vi "updateNonRf.vi"(8 "error in (no error)":errorcluster, 11 "StaticOutputEditor in":refnum<class "StaticOutputEditor.lvclass">) -> (0 "error out":errorcluster, 3 "StaticOutputEditor out":refnum<class "StaticOutputEditor.lvclass">)   [LabVIEW 2011, in "Views.lvlib" / "ScriptEditor.lvlib" / "StaticOutputEditor.lvclass"]
uses:
  StaticOutputEditor.lvclass
  StaticOutputEditor.lvclass/StaticOutputEditor.ctl
  Hal/HWController/HWControllerEvents/HWControllerEvents.lvclass
  Tools/DatabaseHelpers/Database Objects/ChannelArray/ChannelArray.lvclass
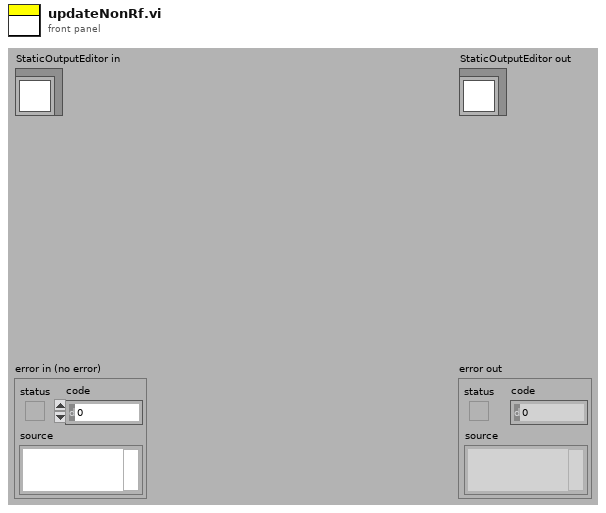
[diagram p1: front panel]
types:
  T1 = enum16{"start", "stop", "statusInquiry", "configure", "resetError", "resourcesInquiry", "reserveResources", "initialise", "resetAllChannels", "staticUpdate", "close", "HWStatus", "error", "resourcesAvailable", "resourcesReserved", "compilerError", "compiledScript", "compilingScript", "runScript", "configureCompiledScript"}
  T2 = cluster{"channelName":string, "value":string, "freq":string, "phase":string}[]
  T3 = cluster{"channelName":string, "value":string, "freq":string, "phase":string}
  T4 = cluster{"incomingEventTypes":cluster{"start":cluster{"Boolean":bool}, "stop":cluster{"Boolean":bool}, "statusInquiry":cluster{"Boolean":bool}, "configure":cluster{"DPScriptPath":path, "TimeStamp":string, "HWLoop?":bool}, "resetError":cluster{"Boolean":bool}, "resourcesInquiry":cluster{"Boolean":bool}, "reserveResources":cluster{"HWList":string[]}, "initialise":cluster{"HWList":string[]}, "close":cluster{"Boolean":bool}, "resetAllChannels":cluster{"Boolean":bool}, "staticChannelUpdate":cluster{"channel_address":string, "calibratedValue":dbl}, "runScript":cluster{"DPScriptPath":path, "TimeStamp":string, "HWLoop?":bool}, "compilingScript":cluster{"Path":path}, "compiledScript":cluster{"Path":path, "timeCompileAt":string}, "compilerError":cluster{"Path":path}, "configureCompiledScript":cluster{"DPScriptPath":path, "TimeStamp":string, "HWLoop?":bool, "CompiledScript":cluster{"ScriptListCompiler.lvclass":refnum<class "ScriptListCompiler.lvclass">, "aoChannels":refnum<class "AnalogOutput.lvclass">[], "doChannels":refnum<class "DigitalOutput.lvclass">[], "rfChannels":refnum<class "DDSOutput.lvclass">[]}}, "restartCompiler":cluster{"restart":bool}, "staticRfChannelUpdate":cluster{"channel_address":string, "Output":cluster{"Frequency(MHz)":dbl, "Amplitude":dbl, "Phase":dbl, "OutputForm":enum16{"Sine", "Square", "Triangle", "Arbitrary"}}}, "cameraUpdate":cluster{"Camera":string, "Type":string, "settings":path}}, "outgoingEventTypes":cluster{"HWStatus":cluster{"status":enum16{"Ready", "Compiling", "Configured", "Running", "Stopping", "Unresolved Error"}}, "error":cluster{"error out":errorcluster}, "resourcesAvailable":cluster{"availableHWList":string[], "reservedHWList":string[]}, "resourcesReserved":cluster{"reservedHWList":string[]}}}
  T5 = cluster{"channel_address":string, "calibratedValue":dbl}
  T6 = cluster{"eventId":enum16{"start", "stop", "statusInquiry", "configure", "resetError", "resourcesInquiry", "reserveResources", "initialise", "resetAllChannels", "staticUpdate", "close", "HWStatus", "error", "resourcesAvailable", "resourcesReserved", "compilerError", "compiledScript", "compilingScript", "runScript", "configureCompiledScript"}, "staticChannelUpdate":cluster{"channel_address":string, "calibratedValue":dbl}}
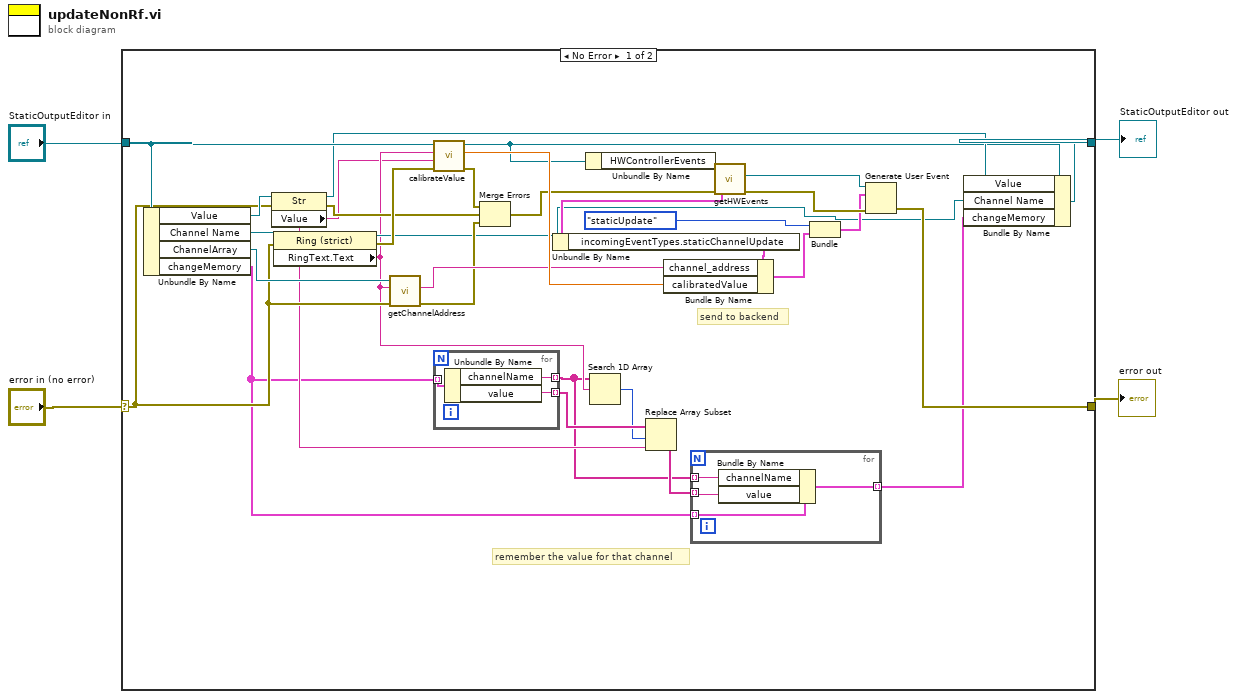
[diagram p0: block diagram]
diagram:
  n1 = case shown="No Error" "error in (no error)" {
    selector: "error in (no error)" -> [w29 w46]
    tunnel: [w37 w46] -> w3
    tunnel: [w14 w45] -> w1
    tunnel: "StaticOutputEditor in" -> [w35 w45]
    frame No Error {
      # "remember the value for that channel"
      # "send to backend"
      n2 = Unbundle By Name(w35) -> ("Value"=w34:refnum<vi>, "Channel Name"=w36:refnum<vi>, "ChannelArray"=w31:refnum<class "ChannelArray.lvclass">, "changeMemory"=w6:T2)
      n3 = property class="Str"(reference=w34, error in=w29) -> (reference out=w17:refnum<vi>, error out=w27:errorcluster, "Value"=w9:string)
      n4 = property class="Ring (strict)"(reference=w36, error in=w29) -> (reference out=w16:refnum<vi>, error out=w32:errorcluster, "RingText.Text"=w12:string)
      n5 = call "getChannelAddress.vi"("error in (no error)"=w29, "channel_name"=w12, "ChannelArray in"=w31) -> ("error out"=w26:errorcluster, "channel_address"=w30:string)  [unwired: 6 in, 1 out]
      n6 = call "calibrateValue.vi"("error in (no error)"=w32, "value"=w9, "channelName"=w12, "StaticOutputEditor in"=w35) -> ("error out"=w28:errorcluster, "calibratedValue"=w33:dbl, "StaticOutputEditor out"=w15:refnum<class "StaticOutputEditor.lvclass">)  [unwired: 5 in]
      n7 = for {
        tunnel: w6 -> [w44] mode=indexing
        tunnel: [w43] -> w7 mode=indexing
        tunnel: [w42] -> w11 mode=indexing
        n8 = Unbundle By Name(w44) -> ("channelName"=w43:string, "value"=w42:string)
      }
      n9 = Merge Errors(w28, w27, w26) -> (w25:errorcluster)
      n10 = Unbundle By Name(w15) -> ("HWControllerEvents"=w24:refnum<class "HWControllerEvents.lvclass">)
      n11 = Search 1D Array(1D array=w7, element=w12) -> (index of element=w10:i32)  [unwired: 1 in]
      n12 = Replace Array Subset(array=w11, new element=w9, index=w10) -> (w8:string[])
      n13 = for {
        tunnel: w8 -> [w39] mode=indexing
        tunnel: w7 -> [w40] mode=indexing
        tunnel: w6 -> [w41] mode=indexing
        tunnel: [w38] -> w5 mode=indexing
        n14 = Bundle By Name(cluster=w41, "channelName"=w40, "value"=w39) -> (w38:T3)
      }
      n15 = call-dynamic "getHWEvents.vi"("error in (no error)"=w25, "HWControllerEvents in"=w24) -> ("error out"=w20:errorcluster, "eventDataTypes"=w23:T4, "HWCEvent"=w18:refnum<user-event>)  [unwired: 6 in, 1 out]
      n16 = Unbundle By Name(w23) -> ("incomingEventTypes.staticChannelUpdate"=w22:T5)
      n17 = Bundle By Name(cluster=w22, "channel_address"=w30, "calibratedValue"=w33) -> (w21:T5)
      n18 = Bundle("eventId"=T1."staticUpdate", "staticChannelUpdate"=w21) -> (w19:T6)  [unwired: 1 in]
      n19 = Generate User Event(user event=w18, event data cluster=w19, error in=w20) -> (error out=w37:errorcluster)  [unwired: 1 out]
      n20 = Bundle By Name(cluster=w15, "Value"=w17, "Channel Name"=w16, "changeMemory"=w5) -> (w14:refnum<class "StaticOutputEditor.lvclass">)
    }
    frame Error {
    }
  }
  "error out" <- w3
  "StaticOutputEditor out" <- w1
